vi "Read AWS Credentials File.vi"(8 "error in (no error)":errorcluster, 11 "Data.S3":refnum<class "LV-Data.S3.lvclass">) -> (0 "error out":errorcluster={"status"=TRUE, "code"=-1, "source"=""}, 2 "AWS Credentials":T1, 3 "Data.S3 out":refnum<class "LV-Data.S3.lvclass">)   [LabVIEW 2019, in "LV-Data.S3.lvclass"]
uses:
  LV-Data.S3.lvclass
  <vilib>/AWS Toolkit/Core/HTTP Request/AWS Credentials.ctl
  LV-Data.S3.lvclass/LV-Data.S3.ctl
  <userlib>/_OpenG.lib/file/file.llb/File Exists - Scalar__ogtk.vi
  <vilib>/AWS Toolkit/Core/HTTP Request/HTTP Request.lvclass
  <vilib>/AWS Toolkit/S3/Bucket/Bucket.lvclass
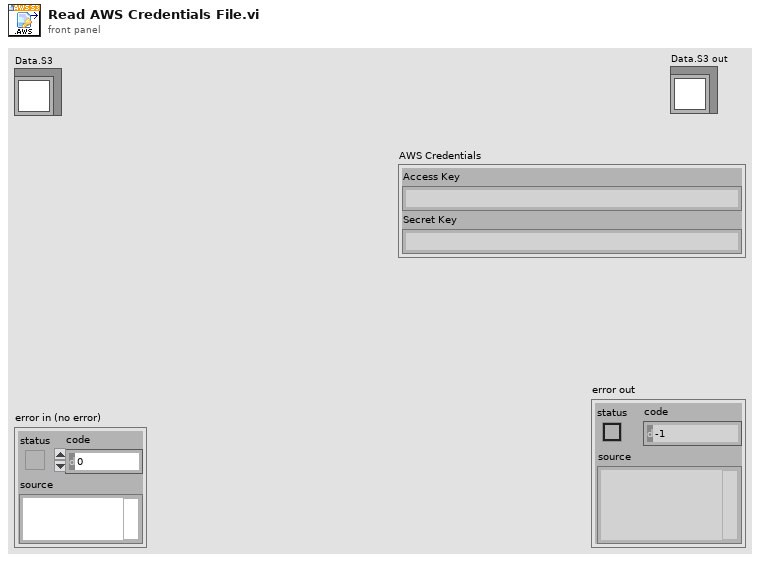
[diagram p1: front panel]
types:
  T1 = typedef "NI_AWS_Core.lvlib/HTTP Request.lvclass/AWS Credentials.ctl" = cluster{"Access Key":string, "Secret Key":string}
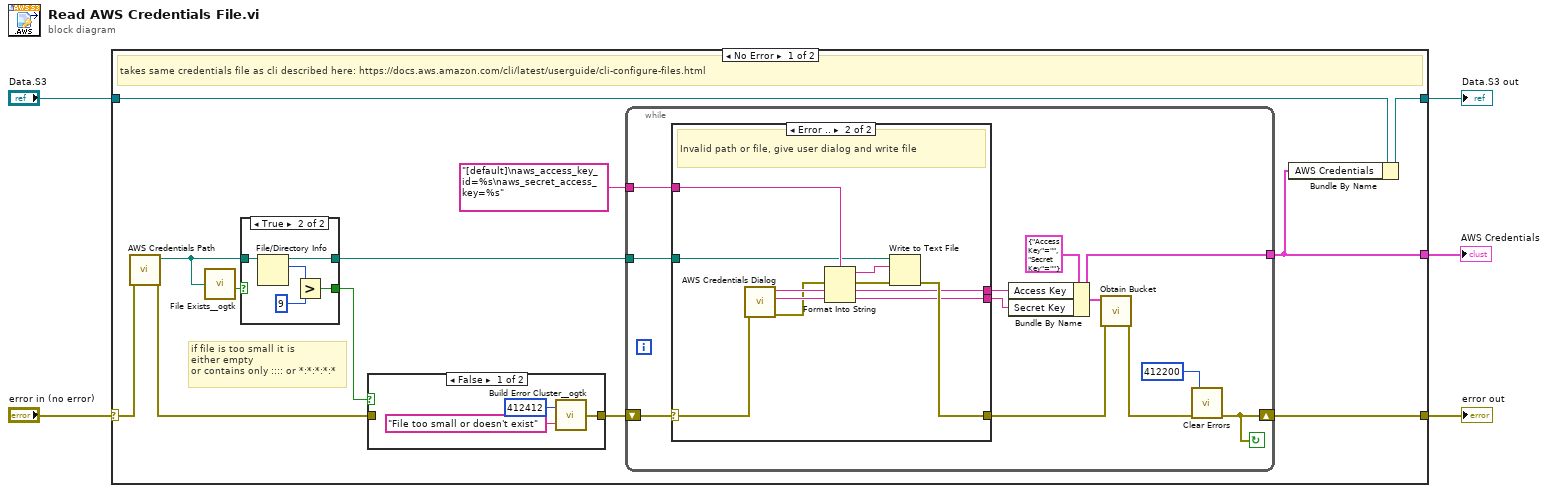
[diagram p0: block diagram]
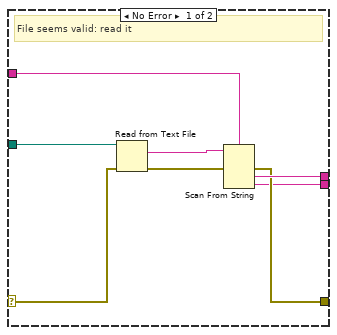
[diagram p3: hidden frame]
diagram:
  n1 = case shown="No Error" "error in (no error)" {
    selector: "error in (no error)" -> [w13 w58]
    tunnel: "Data.S3" -> [w17 w57]
    tunnel: [w16 w57] -> w4
    tunnel: [w14 w58] -> w3
    tunnel: [w9 _] -> w1
    frame No Error {
      # "if file is too small it is\neither empty\nor contains only :::: or *:*:*:*:*"
      # "takes same credentials file as cli described here: https://docs.aws.amazon.com/cli/latest/userguide/cli-configure-files.html"
      n2 = call "AWS Credentials Path.vi"("error in (no error)"=w13) -> ("error out"=w6:errorcluster, "credentials path"=w11:path)  [unwired: 9 in]
      n3 = call-poly <userlib>:"File Exists__ogtk.vi"("file path"=w11) -> ("exists"=w12:bool)  [unwired: 6 in, 1 out]
      n4 = case shown="True" w12 {
        selector: w12 -> [w50 _]
        tunnel: w11 -> [w51 w56]
        tunnel: [w51 w55] -> w10
        tunnel: [w50 w52] -> w8
        frame False {
        }
        frame True {
          n5 = File/Directory Info(path=w56) -> (path out=w55:path, size=w54:i64)  [unwired: 1 in, 5 out]
          n6 = Greater?(x=w54, y=i64 9) -> (0:w52:bool)
        }
      }
      n7 = case shown="False" w8 {
        tunnel: [w18 w21] -> w7
        tunnel: w6 -> [_ w21]
        frame False {
          n8 = call <userlib>:"Build Error Cluster__ogtk.vi"("String to Prepend to source (\"\")"="File too small or doesn't exist" ("String to Prepend to source (\"\")"), "code"=412412) -> ("error out"=w18:errorcluster)
        }
        frame True {
        }
      }
      n9 = while {
        tunnel: "[default]\naws_access_key_id=%s\naws_secret_access_key=%s" ("format string") -> [w31]
        tunnel: w10 -> [w27]
        shift-right: [w23] -> w14
        shift-left: w7 -> [w22]
        tunnel: [w26] -> w9
        stop <- w23 continue-if-true
        n10 = case shown="Error .." w22 {
          selector: w22 -> [w33 w41]
          tunnel: w27 -> [w34 w42]
          tunnel: [w38 w47] -> w28
          tunnel: [w40 w44] -> w30
          tunnel: [w35 w45] -> w29
          tunnel: w31 -> [w36 w46]
          frame No Error {
            # "File seems valid: read it"
            n11 = Read from Text File(file (use dialog)=w34, error in=w33) -> (text=w39:string, error out=w37:errorcluster)  [unwired: 2 in, 2 out]
            n12 = Scan From String(format string=w36, input string=w39, error in=w37) -> (error out=w38:errorcluster, output 1=w40:string, output 2=w35:string)  [unwired: 3 in, 2 out]
          }
          frame Error {
            # "Invalid path or file, give user dialog and write file"
            n13 = call "AWS Credentials Dialog.vi"("error in (no error)"=w41) -> ("error out"=w43:errorcluster, "Secret Access Key"=w45:string, "Access Key ID"=w44:string)  [unwired: 8 in]
            n14 = Format Into String(format string=w46, error in=w43, w44, w45) -> (resulting string=w48:string, error out=w49:errorcluster)  [unwired: 1 in]
            n15 = Write to Text File(file (use dialog)=w42, text=w48, error in=w49) -> (error out=w47:errorcluster)  [unwired: 1 in, 2 out]
          }
        }
        n16 = Bundle By Name(cluster=T1 {"Access Key"="", "Secret Key"=""} ("AWS Credentials"), "Access Key"=w30, "Secret Key"=w29) -> (w26:T1)
        n17 = call <vilib>:"Obtain Bucket.vi"("error in (no error)"=w28, "AWS Credentials"=w26) -> ("error out"=w24:errorcluster)  [unwired: 8 in, 1 out]
        n18 = call <vilib>:"Clear Errors.vi"("error in (no error)"=w24, "specific error code to clear (0: all)"=412200) -> ("error out"=w23:errorcluster)  [unwired: 4 in, 1 out]
      }
      n19 = Bundle By Name(cluster=w17, "AWS Credentials"=w9) -> (w16:refnum<class "LV-Data.S3.lvclass">)
    }
    frame Error {
    }
  }
  "error out" <- w3
  "Data.S3 out" <- w4
  "AWS Credentials" <- w1
